vi "Read Multiple Data.vi"(8 "error in (no error)":errorcluster, 9 "Target":i64=-1, 10 "Target (String)":string, 11 "Hardware Interface in":refnum<class "Hardware Communicator.lvclass">) -> (0 "error out":errorcluster, 1 "1D Integer":i64[](array[numeric]), 2 "1D DBL":dbl[](array[numeric]) format="%#_f", 3 "Hardware Interface out":refnum<class "Hardware Communicator.lvclass">, 4 "Other Type":variant, 5 "Data (String)":string, 6 "Other Type 2":variant)   [LabVIEW 2024, in "Hardware Communicator.lvclass"]
uses:
  Hardware Communicator.lvclass
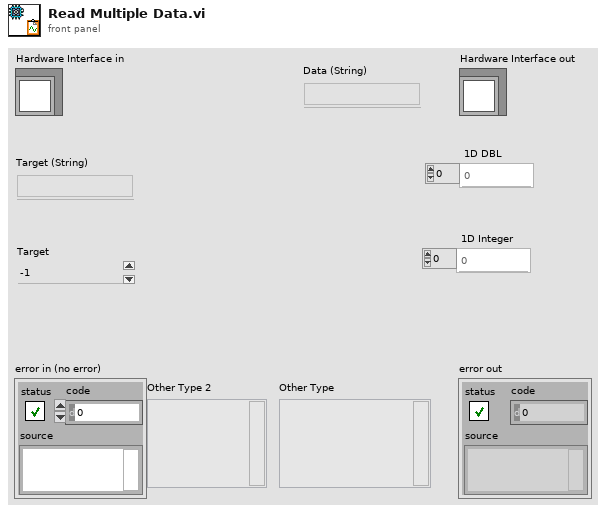
[diagram p1: front panel]
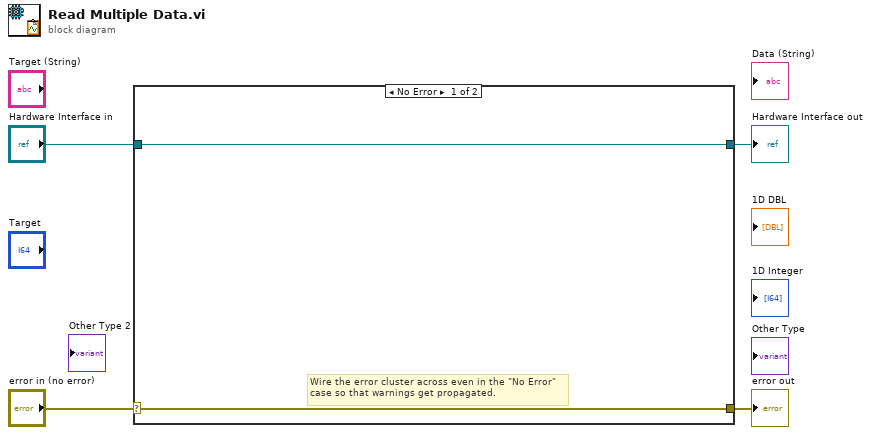
[diagram p0: block diagram]
diagram:
  n1 = case shown="No Error" "error in (no error)" {
    selector: "error in (no error)" -> [w5 w8]
    tunnel: [w5 w8] -> w3
    tunnel: [w6 w7] -> w1
    tunnel: "Hardware Interface in" -> [w6 w7]
    frame No Error {
      # "Wire the error cluster across even in the \"No Error\"\ncase so that warnings get propagated."
    }
    frame Error {
    }
  }
  "error out" <- w3
  "Hardware Interface out" <- w1
